vi "Connect.vi"(8 "error in (no error)":errorcluster, 10 "Serial Setting":T1={"baudRate"=3000000, "parity"=0, "dataBits"=8, "stopBits"=1} {"stopBits" items=["None", "One", "Two", "OnePointFive"]; "parity" items=["None", "Odd", "Even", "Mark", "Space"]}, 11 "LNAX301 in":refnum<class "LNAX301.lvclass">) -> (0 "error out":errorcluster, 1 "SN":string, 3 "LNAX301 out":refnum<class "LNAX301.lvclass">, 4 "COM Port 2":string, 5 "connect":bool)   [LabVIEW 2017, in "LNAX301.lvclass"]
uses:
  LNAX301.lvclass
  <vilib>/Instr/_visa.llb/VISA Find Search Mode.ctl
  DLL/LabVIEW_CSLib.dll
  DLL/Modbus.dll
  LNAX301.lvclass/LNAX301.ctl
panel:
  out "32bit integer":i32[](array[numeric])
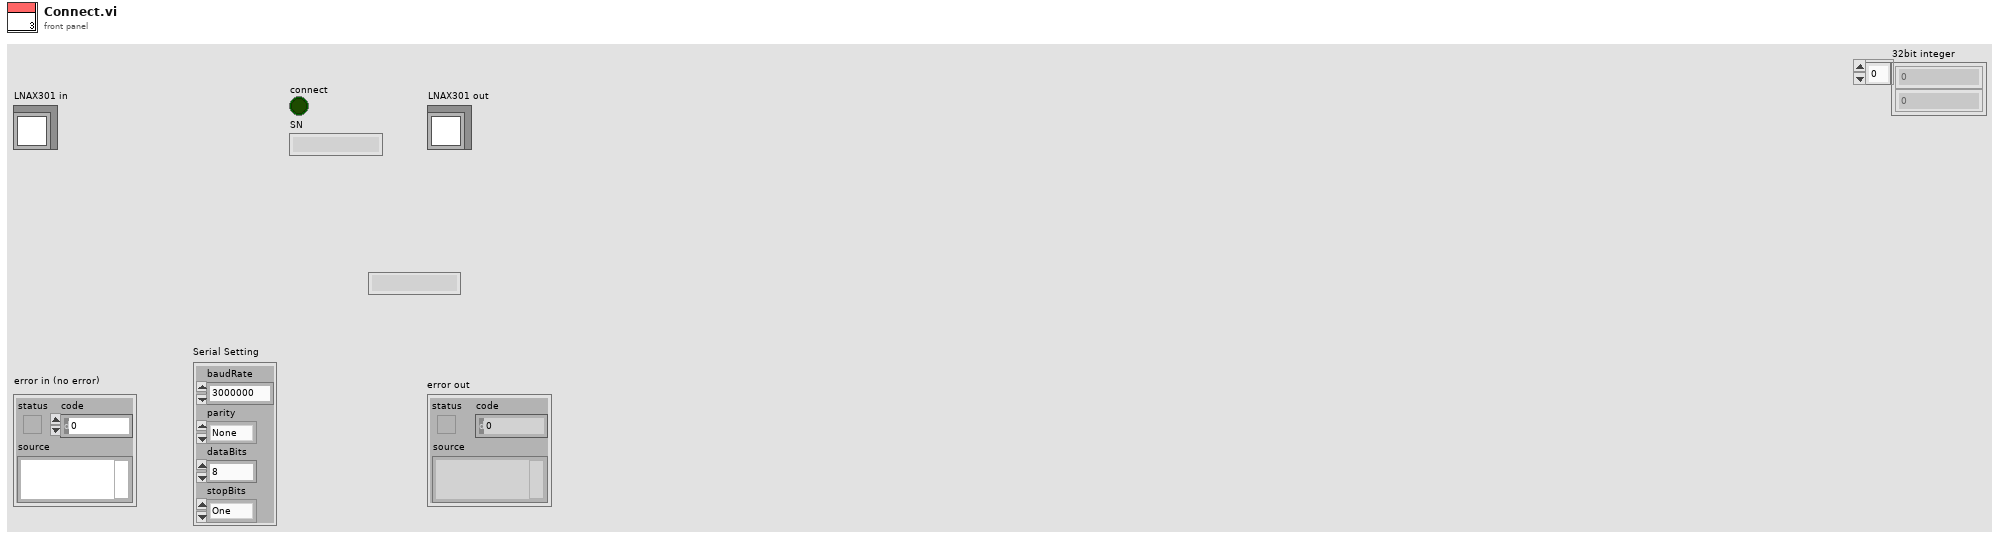
[diagram p1: front panel]
types:
  T1 = cluster{"baudRate":i32, "parity":i32, "dataBits":i32, "stopBits":i32}
  T2 = typedef "VISA Find Search Mode.ctl" = u32
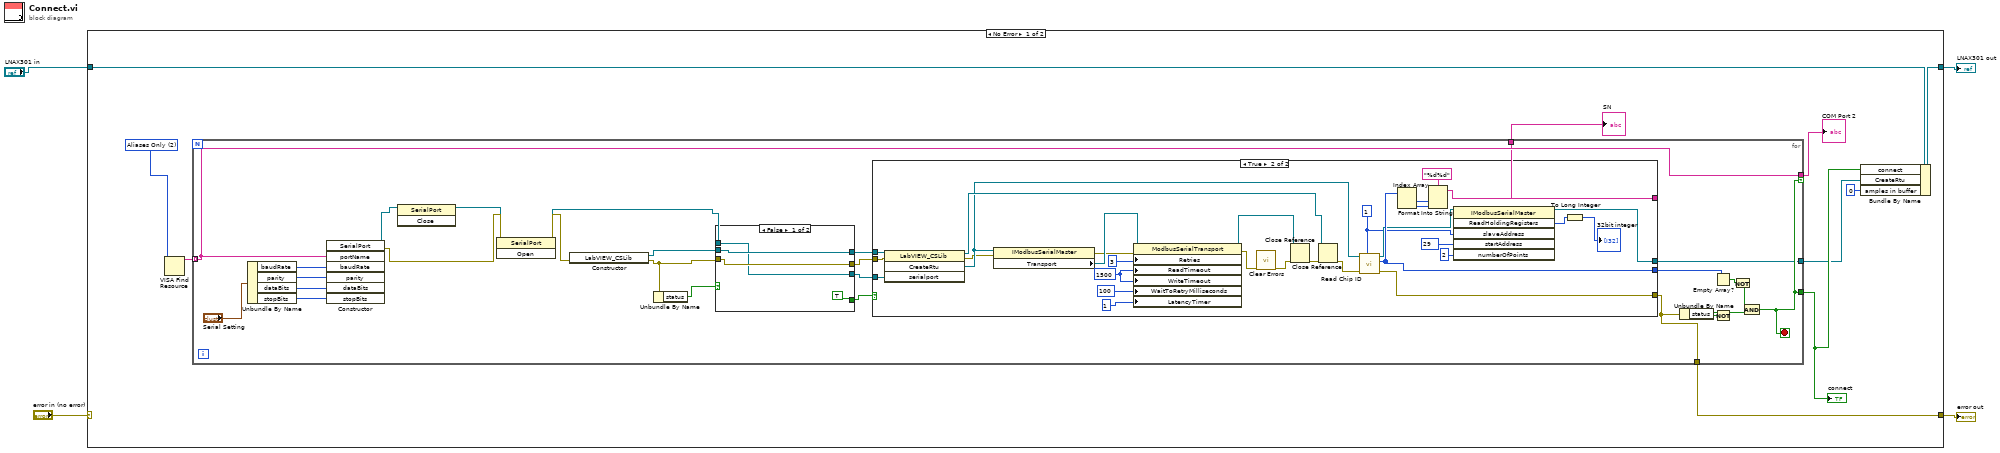
[diagram p0: block diagram]
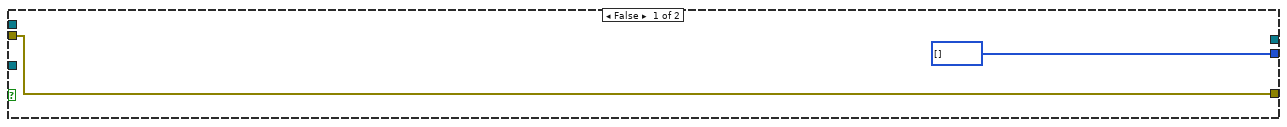
[diagram p2: hidden frame]
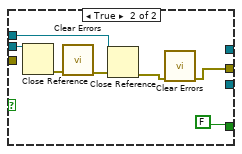
[diagram p3: hidden frame]
diagram:
  n1 = case shown="No Error" "error in (no error)" {
    selector: "error in (no error)" -> [_ w86]
    tunnel: [w9 w86] -> w3
    tunnel: [w13 w85] -> w1
    tunnel: "LNAX301 in" -> [w14 w85]
    frame No Error {
      w12 = T2 2 items=["Canonical Names Only"=0, "Aliases Only"=2, "Include Matching Aliases"=3, "Include All Aliases"=4] ("Search Mode")
      n2 = VISA Find Resource(10:w12) -> (3:w11:string[])  [unwired: 2 in, 2 out]
      n3 = for {
        tunnel: w11 -> [w23] mode=indexing
        tunnel: [w23] -> w7 if=w19
        tunnel: [w19] -> w10
        tunnel: [w18] -> w9
        tunnel: [w16] -> w8
        tunnel: [w15] -> w6
        stop <- w19 stop-if-true
        n4 = Unbundle By Name("Serial Setting") -> ("baudRate"=w40:i32, "parity"=w39:i32, "dataBits"=w38:i32, "stopBits"=w37:i32)
        n5 = constructor class="SerialPort"("portName"=w23, "baudRate"=w40, "parity"=w39, "dataBits"=w38, "stopBits"=w37) -> (reference out=w36:refnum<k24>, error out=w35:errorcluster)  [unwired: 3 in, 6 out]
        n6 = invoke class="SerialPort" method="Close"(reference=w36) -> (reference out=w34:refnum<k24>)  [unwired: 2 in, 2 out]
        n7 = invoke class="SerialPort" method="Open"(reference=w34, error in=w35) -> (reference out=w32:refnum<k24>, error out=w33:errorcluster)  [unwired: 1 in, 1 out]
        n8 = constructor class="LabVIEW_CSLib"(error in=w33) -> (reference out=w29:refnum<k24>, error out=w31:errorcluster)  [unwired: 2 in, 1 out]
        n9 = Unbundle By Name(w31) -> ("status"=w30:bool)
        n10 = case shown="False" w30 {
          tunnel: w29 -> [w77 w84]
          tunnel: [w77 _] -> w28
          tunnel: [w76 w78] -> w27
          tunnel: w31 -> [w76 _]
          tunnel: [TRUE FALSE] -> w17
          tunnel: [w75 _] -> w26
          tunnel: w32 -> [w75 w81]
          frame False {
          }
          frame True {
            n11 = Close Reference(reference=w84) -> (error out=w83:errorcluster)  [unwired: 1 in]
            n12 = call <vilib>:"Clear Errors.vi"("error in (no error)"=w83) -> ("error out"=w80:errorcluster)  [unwired: 5 in, 1 out]
            n13 = Close Reference(reference=w81, error in (no error)=w80) -> (error out=w79:errorcluster)
            n14 = call <vilib>:"Clear Errors.vi"("error in (no error)"=w79) -> ("error out"=w78:errorcluster)  [unwired: 5 in, 1 out]
          }
        }
        n15 = case shown="True" w17 {
          tunnel: w28 -> [_ w73]
          tunnel: w27 -> [w42 w72]
          tunnel: w26 -> [_ w71]
          tunnel: [u16[] [] ("ReadInputRegisters") w55] -> w25
          tunnel: [_ w45] -> w15
          tunnel: [w42 w70] -> w18
          tunnel: [_ w51] -> w16
          frame False {
          }
          frame True {
            w44 = u8 1 ("SlaveID")
            w68 = 1500 ("ReadTimeout")
            n16 = invoke class="LabVIEW_CSLib" method="CreateRtu"(reference=w73, error in=w72, "serialport"=w71) -> (reference out=w64:refnum<k24>, error out=w59:errorcluster, "CreateRtu"=w62:refnum<k24>)  [unwired: 1 in, 1 out]
            n17 = property class="IModbusSerialMaster"(reference=w62, error in=w59) -> (error out=w60:errorcluster, "Transport"=w63:refnum<k24>)  [unwired: 1 out]
            n18 = property class="ModbusSerialTransport"(reference=w63, error in=w60, "Retries"=3, "ReadTimeout"=w68, "WriteTimeout"=w68, "WaitToRetryMilliseconds"=100, "LatencyTimer"=1) -> (reference out=w65:refnum<k24>, error out=w58:errorcluster)
            n19 = call <vilib>:"Clear Errors.vi"("error in (no error)"=w58) -> ("error out"=w57:errorcluster)  [unwired: 5 in, 1 out]
            n20 = Close Reference(reference=w65, error in (no error)=w57) -> (error out=w56:errorcluster)
            n21 = Close Reference(reference=w64, error in (no error)=w56) -> (error out=w61:errorcluster)
            n22 = call "Read Chip ID.vi"("SlaveID"=w44, "error in (no error)"=w61, ".NET Refnum in"=w62) -> ("error out"=w70:errorcluster, "32bit integer"=w55:i32[], ".NET Refnum out"=w46:refnum<k24>)  [unwired: 6 in]
            n23 = Index Array(array=w55) -> (element #1=w54:i32, element #2=w53:i32)  [unwired: 2 in]
            n24 = Format Into String(format string="%d%d", w54, w53) -> (resulting string=w51:string)  [unwired: 2 in, 1 out]
            n25 = invoke class="IModbusSerialMaster" method="ReadHoldingRegisters"(reference=w46, "slaveAddress"=w44, "startAddress"=u16 29, "numberOfPoints"=u16 2) -> (reference out=w45:refnum<k24>, "ReadHoldingRegisters"=w49:u16[])  [unwired: 2 in, 4 out]
            n26 = To Long Integer(number=w49) -> (32bit integer=→"32bit integer":i32[])
          }
        }
        n27 = Unbundle By Name(w18) -> ("status"=w22:bool)
        n28 = Empty Array?(array=w25) -> (empty?=w24:bool)
        n29 = Not(x=w22) -> (.not. x?=w20:bool)
        n30 = Not(x=w24) -> (.not. x?=w21:bool)
        n31 = Compound Arithmetic op=AND(w21, w20) -> (w19:bool)
      }
      "connect" <- w10
      "SN" <- w8
      "COM Port 2" <- w7
      n32 = Bundle By Name(cluster=w14, "connect"=w10, "CreateRtu"=w6, "amples in buffer"=u16 0) -> (w13:refnum<class "LNAX301.lvclass">)
    }
    frame Error {
    }
  }
  "error out" <- w3
  "LNAX301 out" <- w1
